vi "STAGE+mono+counter_edit7.vi"() -> ()   [LabVIEW 2017]
panel:
  out "Spectrum 2":waveform(dbl)(graph)
  in  "Integrating time, 10^-7 sec":dbl=10000000.0
  out "Timeout 2":bool
  in  "scan from":i32=2600
  in  "scan to":i32=4000
  in  "?":bool
  in  "Exit Labview":bool
  in  "step size":dbl=10.0 min=0.0
  in  "?":bool
  out "Spectrum":waveform(dbl)(graph)
  out "Counts":i32
  in  "value (0)":dbl=-9.0
  out "Current WL Wavelength  2":u16 caption="Current Wavelength"
  out "Grt# 2":u8=1 min=1 max=3 step=1
  out "Blaze (nm)":u32=300
  out "Groove/mm":u32=1200
  in  "?":bool
  in  "Channel B Input":u16(ring)=2 items=["Input 1"=1, "Input 2"=2]
  in  "Trigger mode":u16(ring) items=["10 MHz"=0, "Input 2"=2, "Input T"=3]
  out "Current WL Wavelength":u16 caption="Current Wavelength"
  in  "Integrating time, 10^-7 sec":dbl=10000000.0
  in  "gate A mode (CW:0)":i16(slide) scale=0.0..2.0 scale format="%.2f"
  in  "Channel A Input":u16(ring)=1 items=["10 MHz", "Input 1"]
  in  "Time between measurements\n at one point (s)/Dwell Time":dbl=0.002 min=0.002 max=60.0 step=0.001
  in  "Number of Measurements\n to take at one point/ Number of Periods":u16=1 min=1 max=2000 step=1
  in  "Count Mode":u16(ring) items=["A,B for Preset T", "A-B for Preset T", "A+B for Preset T", "A for Preset B"]
  in  "GPIB address":string="23"
  out "Timeout":bool
  out "Serial":u32=12345
  out "Grt#":u8=1 min=1 max=3 step=1
  out "Blaze (nm)":u32=300
  out "Groove/mm":u32=1200
  out "time delay":u32=450000 min=1
  out "Mono port":T1(ring)
  in  "Get position":bool
  out "Position status":dbl format="%.3f"
  in  "Target position":dbl format="%.3f"
  in  "Move":bool
  in  "Motor OFF":bool
  in  "Motor ON":bool
  in  "Step Size [um]":i32=10
  in  "Axis":i32=1
  in  "Rep Rate [Hz]":dbl=500.0
  out "Shots":dbl
  in  "Averaging Time [s]":dbl=0.1
  out "Current Point":i32
  out "Slide":i32(slide) scale=0.0..100.0
  out "Current Position [mm]":dbl
  in  "Axis initial position [mm]":dbl
  out "Axis final Position [mm]":dbl
  in  "Data Points (100 default)":i32=100
  in  "Collect Data!":bool
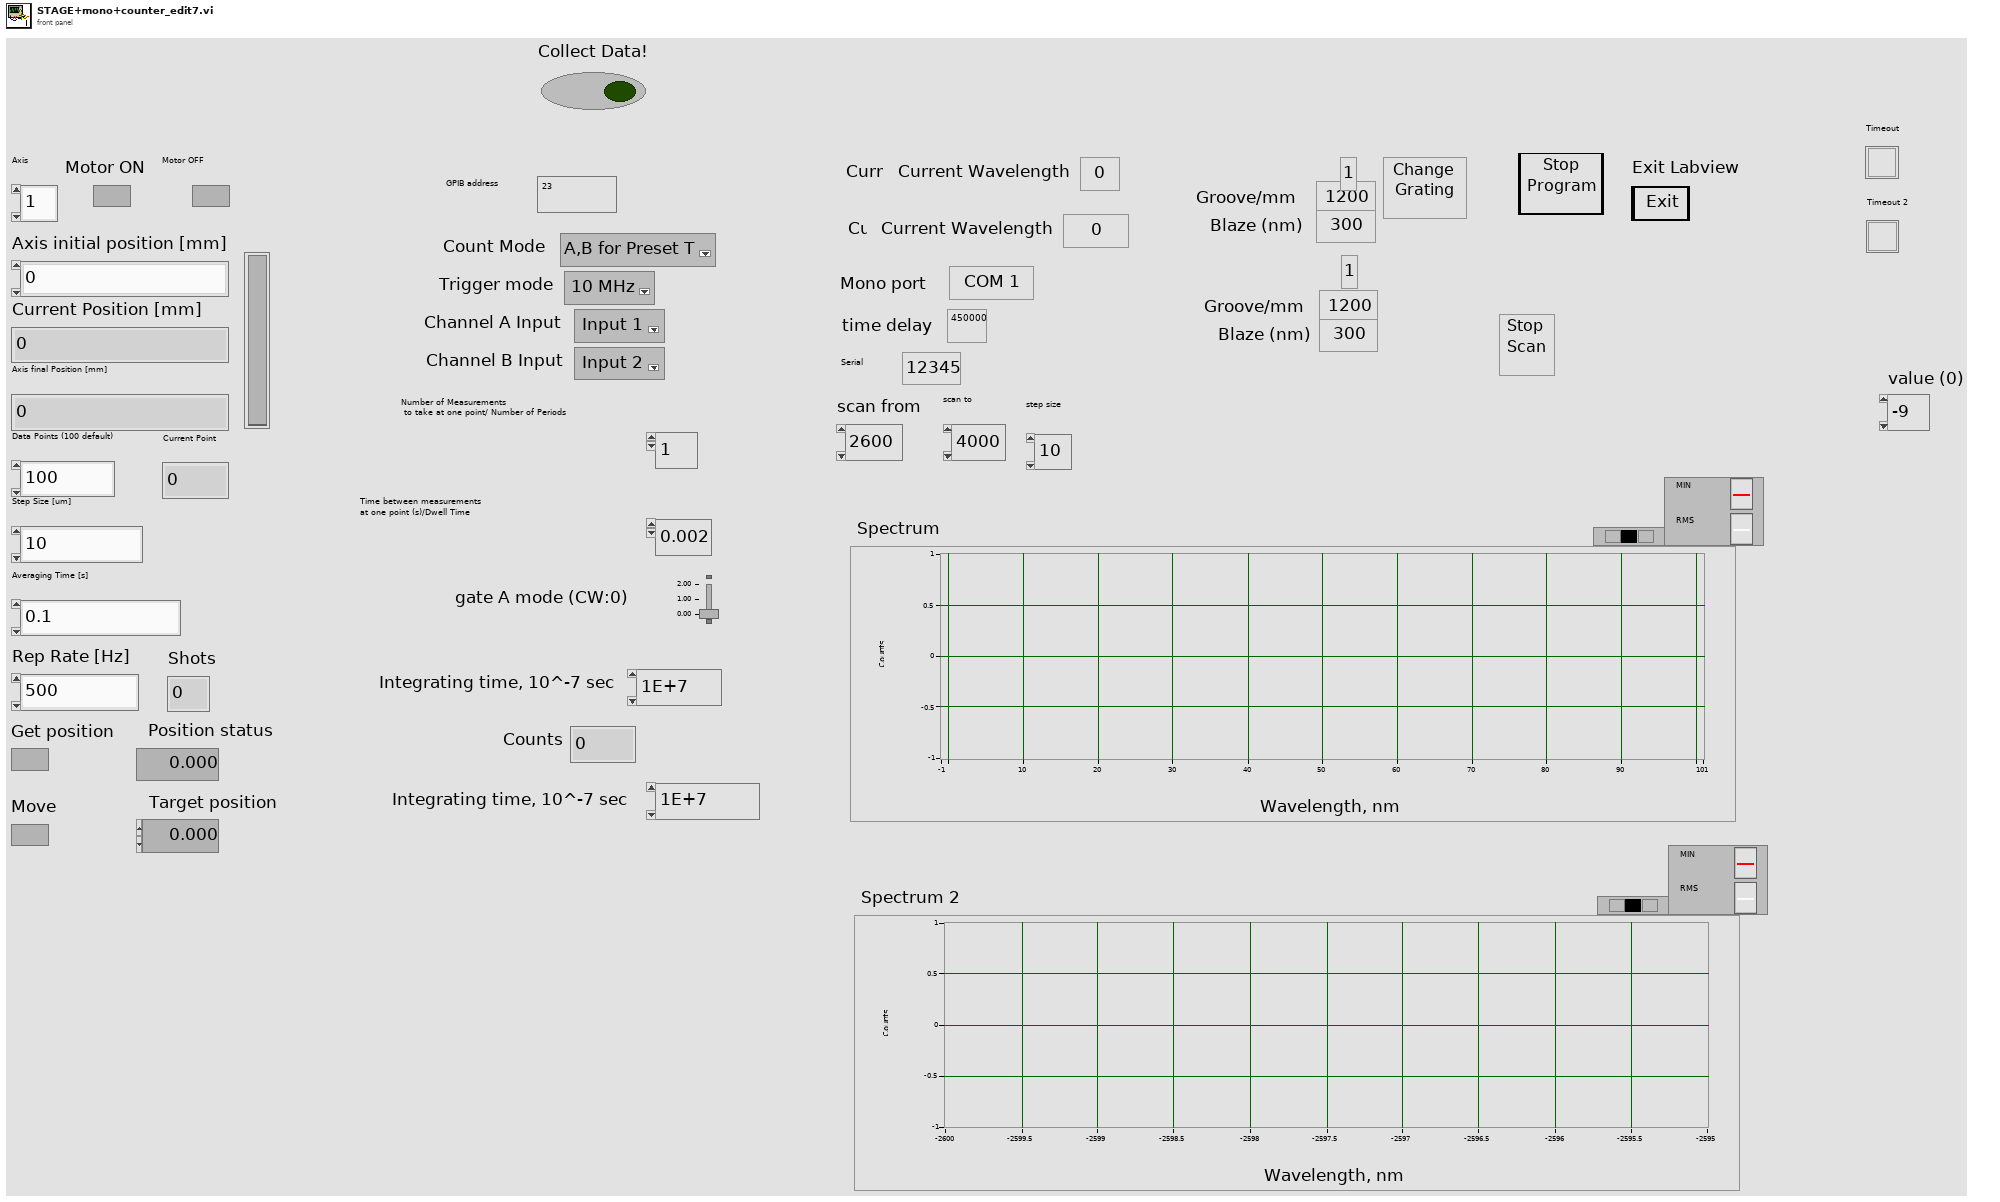
[diagram p1: front panel]
types:
  T1 = enum8{"COM 1", "COM 2", "COM 3", "COM 4", "COM 5", "COM 6", "COM 7", "COM 8", "COM 9"}
  T2 = cluster{"input XON/XOFF":bool, "input HW Handshake":bool, "input alt HW HShk":bool, "output XON/XOFF":bool, "output HW Handshake":bool, "output alt HW HShk":bool, "XOFF byte":u8, "XON byte":u8, "parity error byte":u16}
  T3 = enum16{"no parity", "odd parity", "even parity", "mark parity", "space parity"}
  T4 = cluster{"Y[0]":dbl, "Y[1]":dbl, "Y[2]":dbl, "Y[3]":dbl, "Y[4]":dbl, "Y[5]":dbl, "Y[6]":dbl, "Y[7]":dbl, "Y[8]":dbl}
  T5 = typedef "NI_Matrix.lvlib/RealMatrix.ctl" = dbl[][]
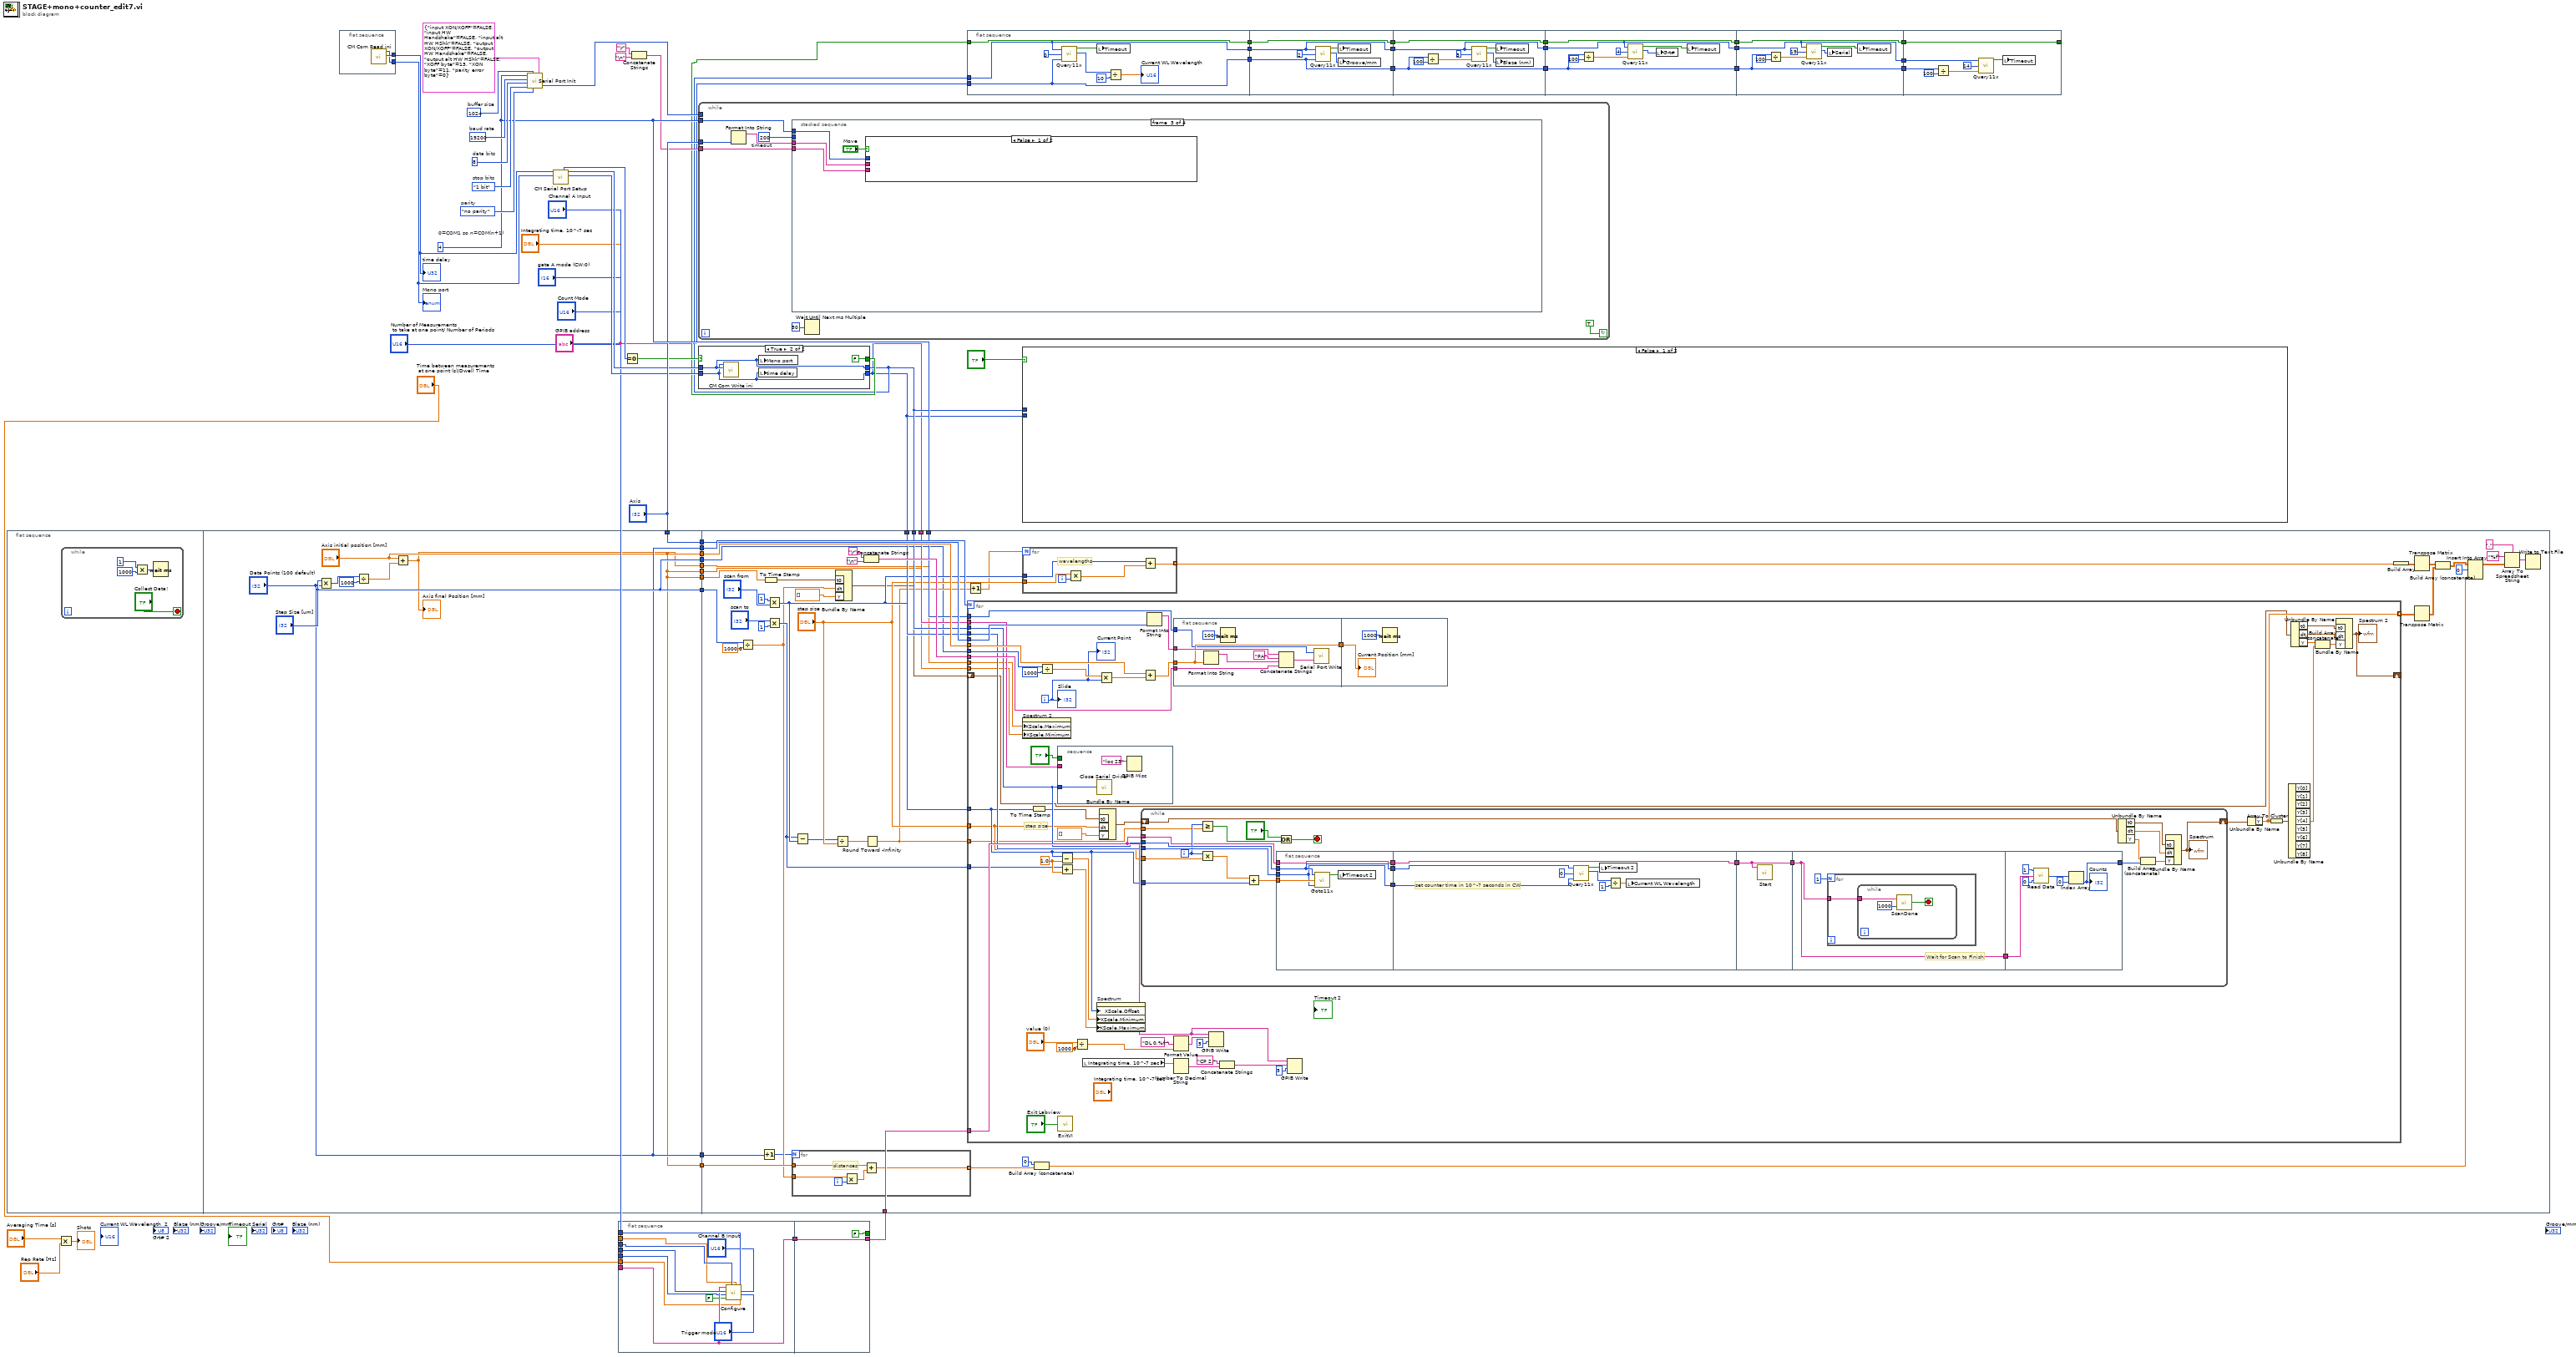
[diagram p0: block diagram]
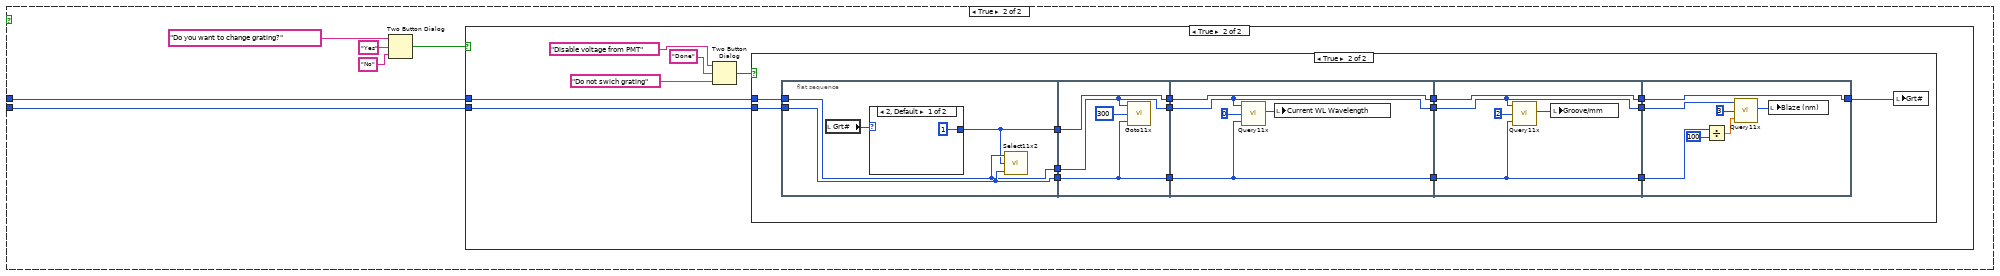
[diagram p2: hidden frame]
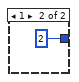
[diagram p5: hidden frame]
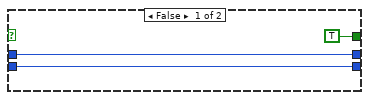
[diagram p6: hidden frame]
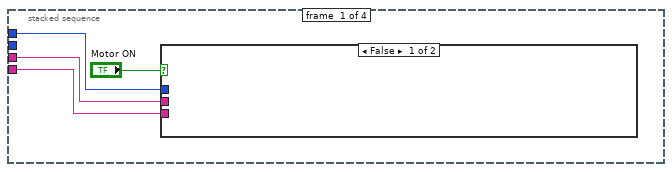
[diagram p7: hidden frame]
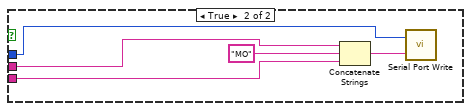
[diagram p8: hidden frame]
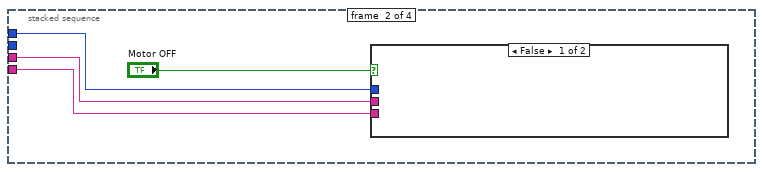
[diagram p9: hidden frame]
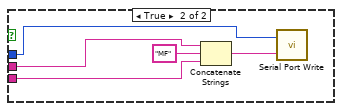
[diagram p10: hidden frame]
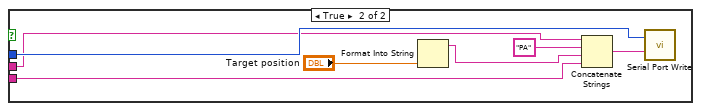
[diagram p11: hidden frame]
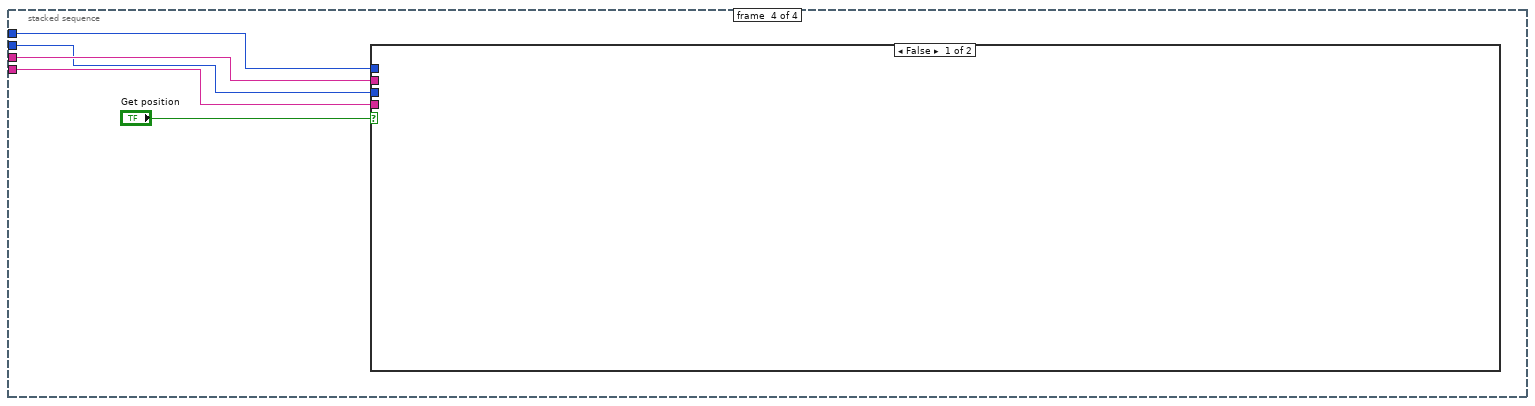
[diagram p12: hidden frame]
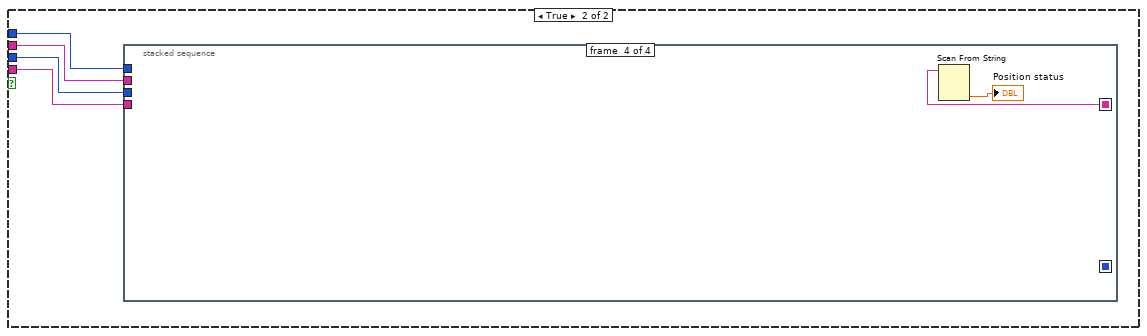
[diagram p13: hidden frame]
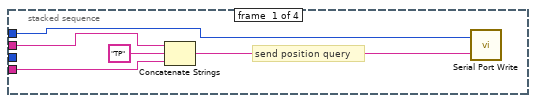
[diagram p14: hidden frame]
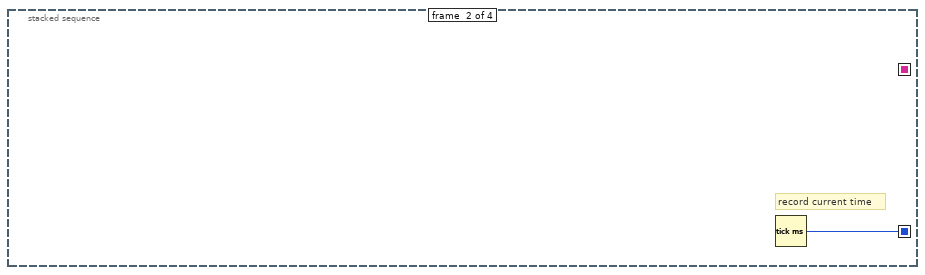
[diagram p15: hidden frame]
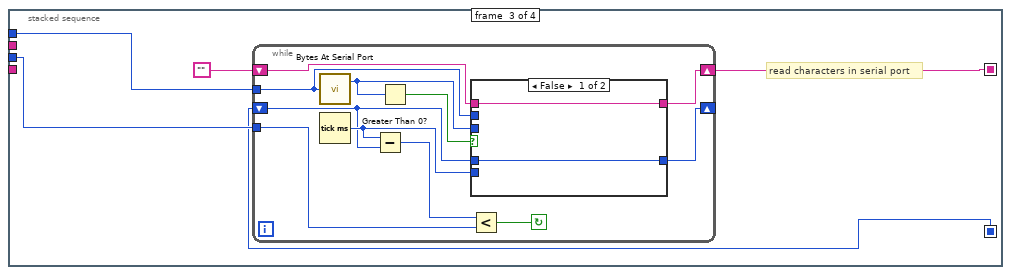
[diagram p16: hidden frame]
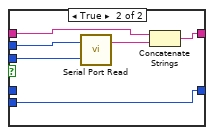
[diagram p17: hidden frame]
diagram:
  w50 = u32 19200  # baud rate
  w49 = u16 8  # data bits
  w48 = enum16{"1 bit", "1.5 bits", "2 bits"}."1 bit"  # stop bits
  w53 = T3."no parity"  # parity
  w47 = 4  # 0=COM1 so n=COM(n+1)
  w52 = u16 1024  # buffer size
  n1 = flat-sequence {
    tunnel: ["Data Points (100 default)"] -> w59
    tunnel: "Axis" -> [w71]
    tunnel: ["Axis initial position [mm]"] -> w58
    tunnel: [w71] -> w57
    tunnel: ["Axis initial position [mm]"] -> w7
    tunnel: ["Step Size [um]"] -> w6
    tunnel: ["Axis initial position [mm]"] -> w5
    tunnel: ["Step Size [um]"] -> w4
    tunnel: ["Data Points (100 default)"] -> w3
    tunnel: ["Axis initial position [mm]"] -> w2
    tunnel: [w64] -> w1
    tunnel: w59 -> [w120]
    tunnel: w58 -> [w119]
    tunnel: w57 -> [w118]
    tunnel: w47 -> [w114]
    tunnel: w11 -> [w113]
    tunnel: w10 -> [w112]
    tunnel: w9 -> [w111]
    tunnel: "GPIB address" -> [w110]
    tunnel: w7 -> [w90]
    tunnel: w6 -> [w89]
    tunnel: w5 -> [w84]
    tunnel: w4 -> [w83]
    tunnel: w3 -> [w80]
    tunnel: w2 -> [w73]
    tunnel: w1 -> [w72]
    frame #0 {
      n2 = while {
        stop <- "Collect Data!" stop-if-true
        n3 = Multiply(x=1, y=1000) -> (x*y=w63:i32)
        n4 = Wait (ms)(milliseconds to wait=w63) -> ()  [unwired: 1 out]
      }
    }
    frame #1 {
      n5 = Multiply(x="Step Size [um]", y="Data Points (100 default)") -> (x*y=w69:i32)
      n6 = Divide(x=w69, y=1000) -> (x/y=w68:dbl)
      n7 = Add(x="Axis initial position [mm]", y=w68) -> (x+y=w64:dbl)
      "Axis final Position [mm]" <- w64
    }
    frame #2 {
      n8 = Divide(x=w89, y=1000.0) -> (x/y=w82:dbl)
      n9 = Increment(x=w80) -> (x+1=w81:i32)
      n10 = To Time Stamp(1:w90) -> (0:w88:timestamp)
      n11 = Multiply(x=1, y="scan from") -> (x*y=w105:i32)
      n12 = Multiply(x="scan to", y=1) -> (x*y=w102:i32)
      n13 = for {
        N: w81 -> [_]
        tunnel: w82 -> [w125]
        tunnel: w84 -> [w123]
        tunnel: [w121] -> w79 mode=indexing
        i -> [w124]
        # "distances"
        n14 = Multiply(x=w125, y=w124) -> (x*y=w122:dbl)
        n15 = Add(x=w123, y=w122) -> (x+y=w121:dbl)
      }
      n16 = Subtract(x=w102, y=w105) -> (x-y=w100:i32)
      n17 = Divide(x=w100, y="step size") -> (x/y=w99:dbl)
      n18 = Bundle By Name("t0"=w88, "dt"=w82, "Y"=dbl[] []) -> (w85:waveform(dbl))  [unwired: 1 in]
      n19 = Concatenate Strings("\r", "\n") -> (w115:string)
      n20 = Round Toward -Infinity(1:w99) -> (0:w98:dbl)
      n21 = for {
        N: w120 -> [_]
        tunnel: w119 -> [w181]
        tunnel: w83 -> [w177]
        tunnel: w118 -> [w174]
        tunnel: w115 -> [w171]
        tunnel: w114 -> [w172]
        tunnel: w113 -> [w169]
        tunnel: w112 -> [w166]
        tunnel: w111 -> [w168]
        tunnel: w110 -> [w167]
        tunnel: [w141] -> w93 mode=indexing
        tunnel: w105 -> [w147]
        tunnel: w102 -> [w146]
        tunnel: "step size" -> [w145]
        tunnel: w98 -> [w144]
        shift-right: [w133] -> _
        shift-left: w85 -> [w137]
        tunnel: w73 -> [w132]
        tunnel: w72 -> [w131]
        i -> [w143]
        w163 = 1.0 ("x")
        # "step size"
        n22 = property on="Spectrum 2" class="WFGraph (strict)"("XScale.Maximum"=w131, "XScale.Minimum"=w132) -> ()  [unwired: 2 in, 2 out]
        n23 = To Time Stamp(1:w147) -> (0:w159:timestamp)
        n24 = Divide(x=w177, y=1000) -> (x/y=w176:dbl)
        n25 = stacked-sequence {
          tunnel: "?" -> [_]
          tunnel: w166 -> [w234]
          tunnel: w167 -> [_]
          frame #0 {
            n26 = call <vilib>:"Close Serial Driver.vi"("port number"=w234) -> ()  [unwired: 1 out]
            n27 = GPIB Misc(0:"loc 23" ("command string")) -> ()  [unwired: 1 in, 3 out]
          }
        }
        n28 = call "ExitVI.vi"("Exit Labview"="Exit Labview") -> ()
        n29 = Subtract(x=w147, y=w163) -> (x-y=w162:dbl)
        n30 = Add(x=w146, y=w163) -> (x+y=w164:dbl)
        n31 = Divide(x="value (0)", y=1000.0) -> (x/y=w148:dbl)
        n32 = local read "Integrating time, 10^-7 sec"() -> (w161:dbl)
        n33 = property on="Spectrum" class="WFGraph (strict)"("XScale.Offset"=w147, "XScale.Minimum"=w162, "XScale.Maximum"=w164) -> ()  [unwired: 2 in, 2 out]
        n34 = Multiply(x=w176, y=w143) -> (x*y=w180:dbl)
        n35 = Bundle By Name("t0"=w159, "dt"=w145, "Y"=dbl[] []) -> (w158:waveform(dbl))  [unwired: 1 in]
        n36 = while {
          tunnel: w166 -> [w205]
          tunnel: w168 -> [w204]
          shift-right: [w194] -> w153
          shift-left: w158 -> [w202]
          tunnel: w169 -> [w193]
          tunnel: w147 -> [w184]
          tunnel: w145 -> [w183]
          tunnel: w144 -> [w182]
          i -> [w199]
          stop <- w203 stop-if-true
          n37 = Greater Or Equal?(x=w199, y=w182) -> (x >= y?=w195:bool)
          n38 = Multiply(x=w199, y=w183) -> (x*y=w206:dbl)
          n39 = Add(x=w206, y=w184) -> (x+y=w185:dbl)
          n40 = flat-sequence {
            tunnel: w185 -> [w211]
            tunnel: w205 -> [w210]
            tunnel: [w210] -> w191
            tunnel: w204 -> [w209]
            tunnel: [w209] -> w190
            tunnel: w193 -> [w207]
            tunnel: [w207] -> w189
            tunnel: w191 -> [w218]
            tunnel: w190 -> [w217]
            tunnel: w189 -> [w215]
            tunnel: [w215] -> w188
            tunnel: w188 -> [w220]
            tunnel: [w220] -> w187
            tunnel: w187 -> [w221]
            tunnel: [w221] -> w186
            tunnel: w186 -> [w228]
            tunnel: [w227] -> w192
            frame #0 {
              n41 = call "Goto11x.vi"("time delay"=w209, "WAVELENGTH"=w211, "port number"=w210) -> ("timeout"=w208:bool)  [unwired: 2 out]
              n42 = local write "Timeout 2"(w208) -> ()
            }
            frame #1 {
              # "set counter time in 10^-7 seconds in CW"
              n43 = call "Query11x.vi"("port number"=w218, "QUERY"=0, "time delay"=w217) -> ("timeout"=w216:bool, "STATUS MESSAGE"=w214:u16)  [unwired: 2 out]
              n44 = local write "Timeout 2"(w216) -> ()
              n45 = Divide(x=w214, y=1) -> (x/y=w213:dbl)
              n46 = local write "Current WL Wavelength"(w213) -> ()
            }
            frame #2 {
              n47 = call "Start.vi"("GPIB Address"=w220) -> ()  [unwired: 9 in]
            }
            frame #3 {
              # "Wait for Scan to Finish"
              n48 = for {
                N: 1 -> [_]
                tunnel: w221 -> [w223]
                n49 = while {
                  tunnel: w223 -> [w224]
                  stop <- w226 stop-if-true
                  n50 = call "ScanDone.vi"("Wait (ms)"=1000, "GPIB Address"=w224) -> ("Scan Finished?"=w226:bool)
                }
              }
            }
            frame #4 {
              n51 = call "Read Data.vi"("Channel Number"=0, "GPIB Address"=w228, "Number of Datapoints"=1) -> ("Data"=w229:i32[])
              n52 = Index Array(array=w229, index=0) -> (element=w227:i32)
              "Counts" <- w227
            }
          }
          n53 = Or(x="?", y=w195) -> (x .or. y?=w203:bool)
          n54 = Unbundle By Name(w202) -> ("t0"=w200:timestamp, "dt"=w201:dbl, "Y"=w198:dbl[])
          n55 = Build Array (concatenate)(w198, w192) -> (w197:dbl[])
          n56 = Bundle By Name("t0"=w200, "dt"=w201, "Y"=w197) -> (w194:waveform(dbl))  [unwired: 1 in]
          "Spectrum" <- w194
        }
        n57 = Add(x=w181, y=w180) -> (x+y=w179:dbl)
        n58 = Format Into String(w174) -> (resulting string=w173:string)  [unwired: 3 in, 1 out]
        n59 = flat-sequence {
          tunnel: w179 -> [w237]
          tunnel: [w237] -> w175
          tunnel: w171 -> [w239]
          tunnel: w173 -> [w238]
          tunnel: w172 -> [w235]
          tunnel: w175 -> [w243]
          frame #0 {
            n60 = Format Into String(w237) -> (resulting string=w236:string)  [unwired: 3 in, 1 out]
            n61 = Wait (ms)(milliseconds to wait=u32 100) -> ()  [unwired: 1 out]
            n62 = Concatenate Strings(w238, "PA" ("Substring"), w236, w239) -> (w241:string)
            n63 = call <vilib>:"Serial Port Write.vi"("string to write"=w241, "port number"=w235) -> ()  [unwired: 1 out]
          }
          frame #1 {
            n64 = Wait (ms)(milliseconds to wait=u32 1000) -> ()  [unwired: 1 out]
            "Current Position [mm]" <- w243
          }
        }
        n65 = Format Value(format string="DL 0,%f;", value (0)=w148) -> (output string=w151:string)  [unwired: 1 in]
        n66 = Number To Decimal String(number=w161) -> (decimal integer string=w156:string)  [unwired: 1 in]
        n67 = GPIB Write(0:w169, 1:w151, 2:i16 5 ("mode (0)")) -> ()  [unwired: 2 in, 2 out]
        n68 = Concatenate Strings("CP 2,", w156) -> (w154:string)
        n69 = GPIB Write(0:w169, 1:w154, 2:i16 5 ("mode (0)")) -> ()  [unwired: 2 in, 2 out]
        n70 = Unbundle By Name(w153) -> ("Y"=w141:dbl[])
        n71 = Array To Cluster(array=w141) -> (cluster=w140:T4)
        n72 = Unbundle By Name(w140) -> ("Y[4]"=w136:dbl)  [unwired: 8 out]
        n73 = Unbundle By Name(w137) -> ("t0"=w139:timestamp, "dt"=w138:dbl, "Y"=w135:dbl[])
        n74 = Build Array (concatenate)(w135, w136) -> (w134:dbl[])
        n75 = Bundle By Name("t0"=w139, "dt"=w138, "Y"=w134) -> (w133:waveform(dbl))  [unwired: 1 in]
        "Spectrum 2" <- w133
        "Current Point" <- w143
        "Slide" <- w143
      }
      n76 = Increment(x=w98) -> (x+1=w97:dbl)
      n77 = for {
        N: w97 -> [_]
        tunnel: "step size" -> [w130]
        tunnel: w105 -> [w128]
        tunnel: [w126] -> w95 mode=indexing
        i -> [w129]
        # "wavelengths"
        n78 = Multiply(x=w130, y=w129) -> (x*y=w127:dbl)
        n79 = Add(x=w128, y=w127) -> (x+y=w126:dbl)
      }
      n80 = Build Array (concatenate)(0, w79) -> (w76:dbl[])
      n81 = Build Array(w95) -> (w94:dbl[][])
      n82 = Transpose Matrix(1:w94) -> (0:w92:dbl[][])
      n83 = Transpose Matrix(1:w93) -> (0:w91:dbl[][])
      n84 = Build Array (concatenate)(w92, w91) -> (w75:T5)
      n85 = Insert Into Array(array=w75, index (row)=0, new element=w76) -> (w74:T5)  [unwired: 1 in]
      n86 = Array To Spreadsheet String(delimiter (Tab)=",", array=w74, 3:"%f" ("format string")) -> (spreadsheet string=w96:string)
      n87 = Write to Text File(text=w96) -> ()  [unwired: 3 in, 3 out]
    }
  }
  n88 = Multiply(x="Averaging Time [s]", y="Rep Rate [Hz]") -> (x*y=→"Shots":dbl)
  n89 = flat-sequence {
    tunnel: [w246] -> w25
    tunnel: [w245] -> w24
    frame #0 {
      n90 = call "CM Com Read ini.vi"() -> ("Mono port"=w245:T1, "time delay1"=w246:u32)  [unwired: 7 in]
    }
  }
  n91 = call <vilib>:"Serial Port Init.vi"("flow control etc."=T2 {"input XON/XOFF"=FALSE, "input HW Handshake"=FALSE, "input alt HW HShk"=FALSE, "output XON/XOFF"=FALSE, "output HW Handshake"=FALSE, "output alt HW HShk"=FALSE, "XOFF byte"=13, "XON byte"=11, "parity error byte"=0}, "parity"=w53, "buffer size"=w52, "stop bits"=w48, "data bits"=w49, "baud rate"=w50, "port number"=w47) -> ("error code"=w46:i32)
  n92 = call "CM Serial Port Setup.vi"("COM port"=w24, "time delay"=w25) -> ("time delay1"=w20:u32, "DK port Out"=w21:T1, "error code"=w23:i32)  [unwired: 7 in]
  n93 = flat-sequence {
    tunnel: "GPIB address" -> [w254]
    tunnel: [w254] -> w26
    tunnel: "Count Mode" -> [w255]
    tunnel: "Number of Measurements\n to take at one point/ Number of Periods" -> [w252]
    tunnel: "Time between measurements\n at one point (s)/Dwell Time" -> [w251]
    tunnel: "Channel A Input" -> [w256]
    tunnel: "gate A mode (CW:0)" -> [w248]
    tunnel: "Integrating time, 10^-7 sec" -> [w247]
    tunnel: w26 -> [w257]
    tunnel: [w257] -> w11
    tunnel: [FALSE] -> _
    frame #0 {
      n94 = call "Configure.vi"("Dwell Time (s)"=w251, "Channel T Input"="Trigger mode", "Channel B Input"="Channel B Input", "Channel A Input"=w256, "Integrating time, 10^-7 sec"=w247, "gate mode (CW:0)"=w248, "Scan End Mode"=FALSE, "Number of Periods"=w252, "Count Mode"=w255, "GPIB Address"=w254) -> ()
    }
    frame #1 {
    }
  }
  n95 = Equal To 0?(x=w23) -> (x = 0?=w22:bool)
  n96 = Concatenate Strings("\r", "\n") -> (w42:string)
  n97 = while {
    tunnel: w47 -> [w261]
    tunnel: w42 -> [w262]
    tunnel: w46 -> [_]
    tunnel: "Axis" -> [w259]
    stop <- TRUE continue-if-true
    w260 = u32 200  # timeout
    n98 = Format Into String(w259) -> (resulting string=w263:string)  [unwired: 3 in, 1 out]
    n99 = stacked-sequence {
      tunnel: w263 -> [w267 w277 w286 w298]
      tunnel: w262 -> [w266 w276 w285 w295]
      tunnel: w261 -> [w268 w278 w287 w297]
      tunnel: w260 -> [_ _ _ w296]
      frame #0 {
        n100 = case shown="False" "Motor ON" {
          tunnel: w268 -> [_ w274]
          tunnel: w267 -> [_ w271]
          tunnel: w266 -> [_ w270]
          frame False {
          }
          frame True {
            n101 = Concatenate Strings(w271, "MO" ("Substring"), w270) -> (w272:string)
            n102 = call <vilib>:"Serial Port Write.vi"("string to write"=w272, "port number"=w274) -> ()  [unwired: 1 out]
          }
        }
      }
      frame #1 {
        n103 = case shown="False" "Motor OFF" {
          tunnel: w278 -> [_ w283]
          tunnel: w277 -> [_ w280]
          tunnel: w276 -> [_ w279]
          frame False {
          }
          frame True {
            n104 = Concatenate Strings(w280, "MF" ("Substring"), w279) -> (w281:string)
            n105 = call <vilib>:"Serial Port Write.vi"("string to write"=w281, "port number"=w283) -> ()  [unwired: 1 out]
          }
        }
      }
      frame #2 {
        n106 = case shown="False" "Move" {
          tunnel: w287 -> [_ w294]
          tunnel: w286 -> [_ w291]
          tunnel: w285 -> [_ w290]
          frame False {
          }
          frame True {
            n107 = Format Into String("Target position") -> (resulting string=w288:string)  [unwired: 3 in, 1 out]
            n108 = Concatenate Strings(w291, "PA" ("Substring"), w288, w290) -> (w292:string)
            n109 = call <vilib>:"Serial Port Write.vi"("string to write"=w292, "port number"=w294) -> ()  [unwired: 1 out]
          }
        }
      }
      frame #3 {
        n110 = case shown="False" "Get position" {
          tunnel: w298 -> [_ w303]
          tunnel: w297 -> [_ w302]
          tunnel: w296 -> [_ w301]
          tunnel: w295 -> [_ w300]
          frame False {
          }
          frame True {
            n111 = stacked-sequence {
              seq-local: [_ w309 _ _] -> [_ _ w311 _]
              seq-local: [_ _ w310 _] -> [_ _ _ w335]
              tunnel: w303 -> [w306 _ _ _]
              tunnel: w302 -> [w305 _ w314 _]
              tunnel: w301 -> [_ _ w312 _]
              tunnel: w300 -> [w304 _ _ _]
              frame #0 {
                # "send position query"
                n112 = Concatenate Strings(w306, "TP" ("Substring"), w304) -> (w307:string)
                n113 = call <vilib>:"Serial Port Write.vi"("string to write"=w307, "port number"=w305) -> ()  [unwired: 1 out]
              }
              frame #1 {
                # "record current time"
                n114 = Tick Count (ms)() -> (millisecond timer value=w309:u32)
              }
              frame #2 {
                # "read characters in serial port"
                n115 = while {
                  shift-left: w311 -> [w315]
                  shift-right: [w316] -> _
                  tunnel: w312 -> [w319]
                  shift-left: "" -> [w322]
                  shift-right: [w321] -> w310
                  tunnel: w314 -> [w323]
                  stop <- w318 continue-if-true
                  n116 = call <vilib>:"Bytes At Serial Port.vi"("port number"=w323) -> ("byte count"=w324:u32)  [unwired: 1 out]
                  n117 = Tick Count (ms)() -> (millisecond timer value=w317:u32)
                  n118 = Subtract(x=w317, y=w315) -> (x-y=w320:u32)
                  n119 = Greater Than 0?(x=w324) -> (x > 0?=w325:bool)
                  n120 = case shown="False" w325 {
                    tunnel: w324 -> [_ w333]
                    tunnel: w323 -> [_ w332]
                    tunnel: w322 -> [w327 w330]
                    tunnel: [w327 w329] -> w321
                    tunnel: [w326 w328] -> w316
                    tunnel: w317 -> [_ w328]
                    tunnel: w315 -> [w326 _]
                    frame False {
                    }
                    frame True {
                      n121 = call <vilib>:"Serial Port Read.vi"("requested byte count"=w333, "port number"=w332) -> ("string read"=w331:string)  [unwired: 1 out]
                      n122 = Concatenate Strings(w330, w331) -> (w329:string)
                    }
                  }
                  n123 = Less?(x=w320, y=w319) -> (x < y?=w318:bool)
                }
              }
              frame #3 {
                n124 = Scan From String(input string=w335) -> (output 1=→"Position status":dbl)  [unwired: 4 in, 3 out]
              }
            }
          }
        }
      }
    }
    n125 = Wait Until Next ms Multiple(millisecond multiple=u32 50) -> ()  [unwired: 1 out]
  }
  n126 = case shown="True" w22 {
    tunnel: w21 -> [w338 w341]
    tunnel: w20 -> [w337 w340]
    tunnel: [w338 w341] -> w10
    tunnel: [w337 w340] -> w9
    tunnel: [TRUE FALSE] -> w19
    frame False {
    }
    frame True {
      n127 = call "CM Com Write ini.vi"("time delay1"=w341, "Mono port"=w340) -> ()  [unwired: 7 in]
      n128 = local write "Mono port"(w341) -> ()
      n129 = local write "time delay"(w340) -> ()
    }
  }
  n130 = flat-sequence {
    tunnel: w9 -> [w347]
    tunnel: [w347] -> w41
    tunnel: w10 -> [w349]
    tunnel: [w349] -> w40
    tunnel: w19 -> [w345]
    tunnel: [w345] -> w39
    tunnel: w41 -> [w352]
    tunnel: [w352] -> w38
    tunnel: w40 -> [w354]
    tunnel: [w354] -> w37
    tunnel: w39 -> [w350]
    tunnel: [w350] -> w36
    tunnel: w38 -> [w362]
    tunnel: [w362] -> w35
    tunnel: w37 -> [w359]
    tunnel: [w359] -> w34
    tunnel: w36 -> [w356]
    tunnel: [w356] -> w33
    tunnel: w35 -> [w370]
    tunnel: [w370] -> w32
    tunnel: w34 -> [w367]
    tunnel: [w367] -> w31
    tunnel: w33 -> [w364]
    tunnel: [w364] -> w30
    tunnel: w32 -> [w378]
    tunnel: [w378] -> w29
    tunnel: w31 -> [w375]
    tunnel: [w375] -> w28
    tunnel: w30 -> [w372]
    tunnel: [w372] -> w27
    tunnel: w29 -> [w385]
    tunnel: w28 -> [w382]
    tunnel: [w380] -> _
    tunnel: w27 -> [w380]
    frame #0 {
      n131 = call "Query11x.vi"("port number"=w349, "QUERY"=u16 0, "time delay"=w347) -> ("timeout"=w346:bool, "STATUS MESSAGE"=w344:u16)  [unwired: 2 out]
      n132 = local write "Timeout"(w346) -> ()
      n133 = Divide(x=w344, y=10 ("Numeric")) -> (x/y=→"Current WL Wavelength":dbl)
    }
    frame #1 {
      n134 = call "Query11x.vi"("port number"=w354, "QUERY"=u16 2, "time delay"=w352) -> ("timeout"=w351:bool, "STATUS MESSAGE"=w353:u16)  [unwired: 2 out]
      n135 = local write "Timeout"(w351) -> ()
      n136 = local write "Groove/mm"(w353) -> ()
    }
    frame #2 {
      n137 = Divide(x=w362, y=i16 100 ("device (1)")) -> (x/y=w360:dbl)
      n138 = call "Query11x.vi"("port number"=w359, "QUERY"=u16 3, "time delay"=w360) -> ("timeout"=w357:bool, "STATUS MESSAGE"=w358:u16)  [unwired: 2 out]
      n139 = local write "Timeout"(w357) -> ()
      n140 = local write "Blaze (nm)"(w358) -> ()
    }
    frame #3 {
      n141 = Divide(x=w370, y=i16 100 ("device (1)")) -> (x/y=w368:dbl)
      n142 = call "Query11x.vi"("port number"=w367, "QUERY"=u16 4, "time delay"=w368) -> ("timeout"=w365:bool, "STATUS MESSAGE"=w366:u16)  [unwired: 2 out]
      n143 = local write "Grt#"(w366) -> ()
      n144 = local write "Timeout"(w365) -> ()
    }
    frame #4 {
      n145 = Divide(x=w378, y=i16 100 ("device (1)")) -> (x/y=w376:dbl)
      n146 = call "Query11x.vi"("port number"=w375, "QUERY"=u16 19, "time delay"=w376) -> ("timeout"=w373:bool, "STATUS MESSAGE"=w374:u16)  [unwired: 2 out]
      n147 = local write "Serial"(w374) -> ()
      n148 = local write "Timeout"(w373) -> ()
    }
    frame #5 {
      n149 = Divide(x=w385, y=i16 100 ("device (1)")) -> (x/y=w383:dbl)
      n150 = call "Query11x.vi"("port number"=w382, "QUERY"=u16 14, "time delay"=w383) -> ("timeout"=w381:bool)  [unwired: 3 out]
      n151 = local write "Timeout"(w381) -> ()
    }
  }
  n152 = case shown="False" "?" {
    tunnel: w9 -> [_ w388]
    tunnel: w10 -> [_ w387]
    frame False {
    }
    frame True {
      n153 = Two Button Dialog(message="Do you want to change grating?", 1:"No" ("F button name (\"Cancel\")"), 2:"Yes" ("T button name (\"OK\")")) -> (T button?=w389:bool)
      n154 = case shown="True" w389 {
        tunnel: w388 -> [_ w394]
        tunnel: w387 -> [_ w393]
        frame False {
        }
        frame True {
          n155 = Two Button Dialog(message="Disable voltage from PMT", 1:"Do not swich grating" ("F button name (\"Cancel\")"), 2:"Done" ("T button name (\"OK\")")) -> (T button?=w395:bool)
          n156 = case shown="True" w395 {
            tunnel: w394 -> [_ w413]
            tunnel: w393 -> [_ w412]
            frame False {
            }
            frame True {
              n157 = flat-sequence {
                tunnel: w413 -> [w417]
                tunnel: [w417] -> w410
                tunnel: w412 -> [w416]
                tunnel: [w416] -> w409
                tunnel: [w414] -> w408
                tunnel: w410 -> [w421]
                tunnel: [w421] -> w407
                tunnel: w409 -> [w422]
                tunnel: [w422] -> w406
                tunnel: w408 -> [w420]
                tunnel: [w420] -> w405
                tunnel: w407 -> [w428]
                tunnel: [w428] -> w404
                tunnel: w406 -> [w427]
                tunnel: [w427] -> w403
                tunnel: w405 -> [w424]
                tunnel: [w424] -> w402
                tunnel: w404 -> [w431]
                tunnel: [w431] -> w401
                tunnel: w403 -> [w432]
                tunnel: [w432] -> w400
                tunnel: w402 -> [w429]
                tunnel: [w429] -> w399
                tunnel: w401 -> [w436]
                tunnel: w400 -> [w437]
                tunnel: [w434] -> w411
                tunnel: w399 -> [w434]
                frame #0 {
                  n158 = local read "Grt#"() -> (w415:u8)
                  n159 = case shown="2, Default" w415 {
                    tunnel: [1 2] -> w414
                    frame 2, Default {
                    }
                    frame 1 {
                    }
                  }
                  n160 = call "Select11x2.vi"("time delay"=w417, "NEW GRT?"=w414, "port number"=w416) -> ()  [unwired: 3 out]
                }
                frame #1 {
                  n161 = call "Goto11x.vi"("time delay"=w421, "WAVELENGTH"=u16 300, "port number"=w422) -> ()  [unwired: 3 out]
                }
                frame #2 {
                  n162 = call "Query11x.vi"("port number"=w427, "QUERY"=u16 0, "time delay"=w428) -> ("STATUS MESSAGE"=w425:u16)  [unwired: 3 out]
                  n163 = local write "Current WL Wavelength"(w425) -> ()
                }
                frame #3 {
                  n164 = call "Query11x.vi"("port number"=w432, "QUERY"=u16 2, "time delay"=w431) -> ("STATUS MESSAGE"=w430:u16)  [unwired: 3 out]
                  n165 = local write "Groove/mm"(w430) -> ()
                }
                frame #4 {
                  n166 = Divide(x=w436, y=i16 100 ("device (1)")) -> (x/y=w438:dbl)
                  n167 = call "Query11x.vi"("port number"=w437, "QUERY"=u16 3, "time delay"=w438) -> ("STATUS MESSAGE"=w435:u16)  [unwired: 3 out]
                  n168 = local write "Blaze (nm)"(w435) -> ()
                }
              }
              n169 = local write "Grt#"(w411) -> ()
            }
          }
        }
      }
    }
  }
  "Mono port" <- w24
  "time delay" <- w25
